vi "green_speedgate.vi"(4 "sat":cluster{"Lower value":i32, "Upper value":i32}={"Lower value"=30, "Upper value"=138}, 5 "luma":cluster{"Lower value":i32, "Upper value":i32}={"Lower value"=37, "Upper value"=106}, 6 "hue":cluster{"Lower value":i32, "Upper value":i32}={"Lower value"=80, "Upper value"=131}, 8 "error in (no error)":errorcluster, 11 "Image Src":T1) -> (0 "error out":errorcluster, 1 "max":dbl[](array[numeric]), 2 "green particles":dbl[][](array[numeric]), 3 "Image Out":T1(plugin-control))   [LabVIEW 2009]
uses:
  <vilib>/vision/Image Controls.llb/IMAQ Image.ctl
  <vilib>/vision/NI_Vision_Development_Module.lvlib
panel:
  out "Array":dbl[](array[numeric])
  out "Particle Measurements (Pixels)":dbl[][](array[numeric]) format="%.2f"
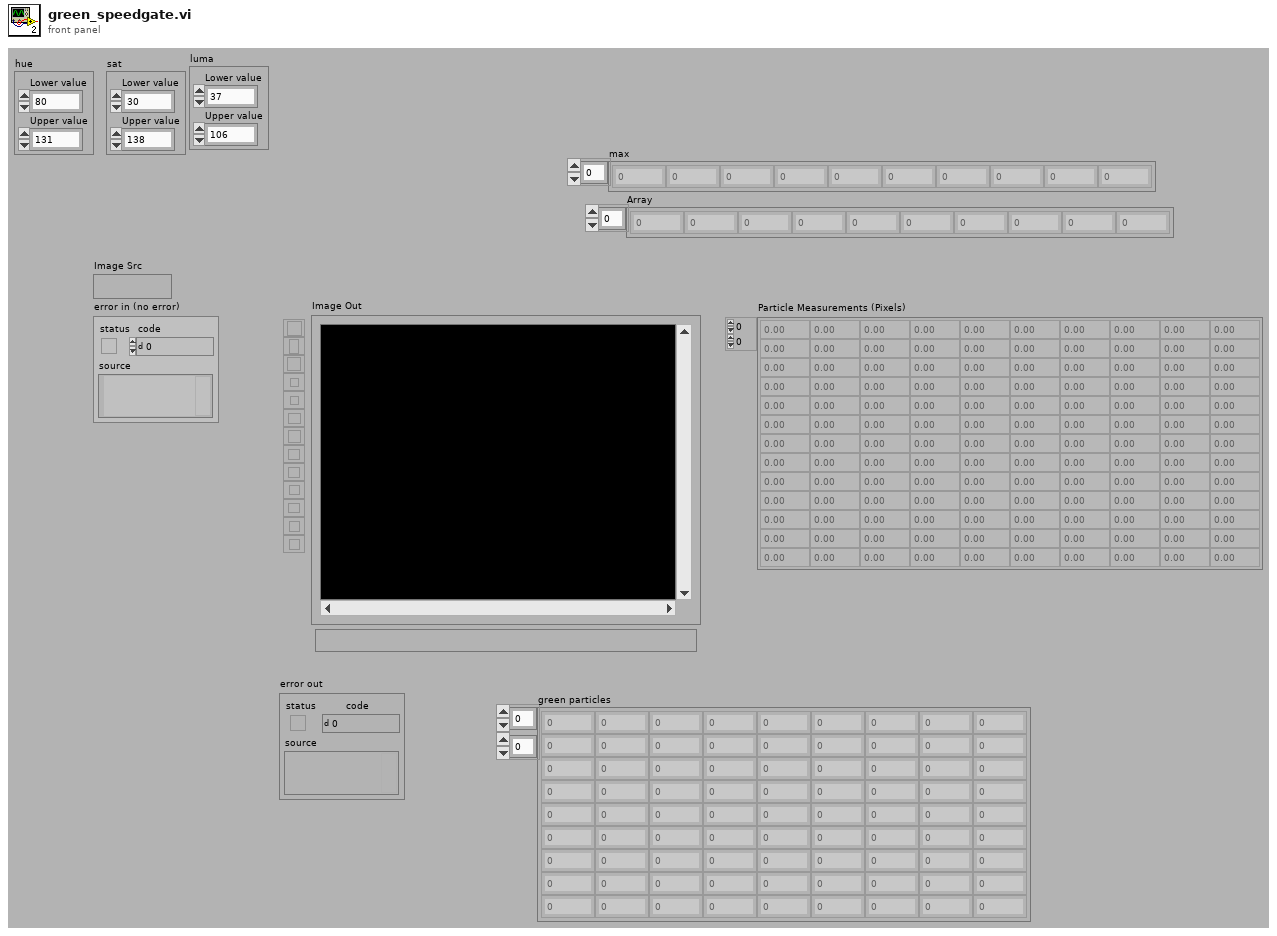
[diagram p1: front panel]
types:
  T1 = typedef "IMAQ Image.ctl" = refnum<image>
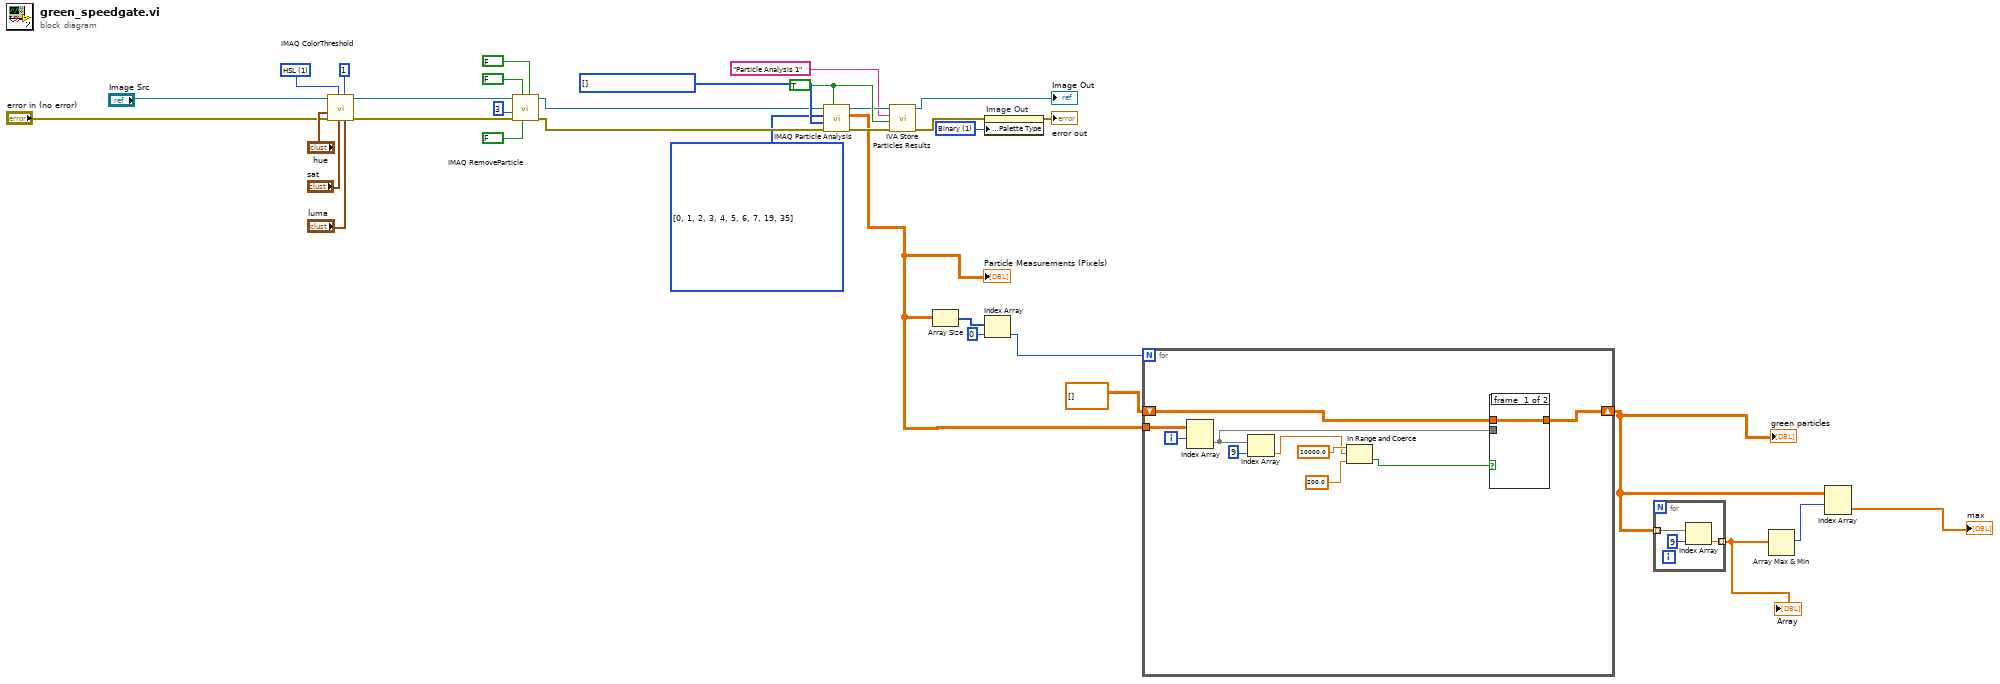
[diagram p0: block diagram]
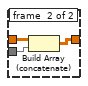
[diagram p2: hidden frame]
diagram:
  w19 = i32[] [] items=["Center of Mass X", "Center of Mass Y", "First Pixel X", "First Pixel Y", "Bounding Rect Left", "Bounding Rect Top", "Bounding Rect Right", "Bounding Rect Bottom", "Max Feret Diameter Start X", "Max Feret Diameter Start Y", "Max Feret Diameter End X", "Max Feret Diameter End Y", "Max Horiz. Segment Length Left", "Max Horiz. Segment Length Right", "Max Horiz. Segment Length Row", "-", "Bounding Rect Width", "Bounding Rect Height", "Bounding Rect Diagonal", "Perimeter", "Convex Hull Perimeter", "Holes' Perimeter", "Max Feret Diameter", "Equivalent Ellipse Major Axis", "Equivalent Ellipse Minor Axis", "Equivalent Ellipse Minor Axis (Feret)", "Equivalent Rect Long Side", "Equivalent Rect Short Side", "Equivalent Rect Diagonal", "Equivalent Rect Short Side (Feret)", "Average Horiz. Segment Length", "Average Vert. Segment Length", "Hydraulic Radius", "Waddel Disk Diameter", "-", "Area", "Holes' Area", "Particle & Holes' Area", "Convex Hull Area", "Image Area", "-", "Number of Holes", "Number of Horiz. Segments", "Number of Vert. Segments", "-", "Orientation", "Max Feret Diameter Orientation", "-", "% Area/Image Area", "% Area/(Particle & Holes' Area)", "Ratio of Equivalent Ellipse Axes", "Ratio of Equivalent Rect Sides", "-", "Elongation Factor", "Compactness Factor", "Heywood Circularity Factor", "Type Factor", "-", "Sum X", "Sum Y", "Sum XX", "Sum XY", "Sum YY", "Sum XXX", "Sum XXY", "Sum XYY", "Sum YYY", "-", "Moment of Inertia XX", "Moment of Inertia XY", "Moment of Inertia YY", "Moment of Inertia XXX", "Moment of Inertia XXY", "Moment of Inertia XYY", "Moment of Inertia YYY", "Norm. Moment of Inertia XX", "Norm. Moment of Inertia XY", "Norm. Moment of Inertia YY", "Norm. Moment of Inertia XXX", "Norm. Moment of Inertia XXY", "Norm. Moment of Inertia XYY", "Norm. Moment of Inertia YYY", "Hu Moment 1", "Hu Moment 2", "Hu Moment 3", "Hu Moment 4", "Hu Moment 5", "Hu Moment 6", "Hu Moment 7"] ("Real-World Measurements")
  w12 = i32[] [0, 1, 2, 3, 4, 5, 6, 7, 19, 35] items=["Center of Mass X", "Center of Mass Y", "First Pixel X", "First Pixel Y", "Bounding Rect Left", "Bounding Rect Top", "Bounding Rect Right", "Bounding Rect Bottom", "Max Feret Diameter Start X", "Max Feret Diameter Start Y", "Max Feret Diameter End X", "Max Feret Diameter End Y", "Max Horiz. Segment Length Left", "Max Horiz. Segment Length Right", "Max Horiz. Segment Length Row", "-", "Bounding Rect Width", "Bounding Rect Height", "Bounding Rect Diagonal", "Perimeter", "Convex Hull Perimeter", "Holes' Perimeter", "Max Feret Diameter", "Equivalent Ellipse Major Axis", "Equivalent Ellipse Minor Axis", "Equivalent Ellipse Minor Axis (Feret)", "Equivalent Rect Long Side", "Equivalent Rect Short Side", "Equivalent Rect Diagonal", "Equivalent Rect Short Side (Feret)", "Average Horiz. Segment Length", "Average Vert. Segment Length", "Hydraulic Radius", "Waddel Disk Diameter", "-", "Area", "Holes' Area", "Particle & Holes' Area", "Convex Hull Area", "Image Area", "-", "Number of Holes", "Number of Horiz. Segments", "Number of Vert. Segments", "-", "Orientation", "Max Feret Diameter Orientation", "-", "% Area/Image Area", "% Area/(Particle & Holes' Area)", "Ratio of Equivalent Ellipse Axes", "Ratio of Equivalent Rect Sides", "-", "Elongation Factor", "Compactness Factor", "Heywood Circularity Factor", "Type Factor", "-", "Sum X", "Sum Y", "Sum XX", "Sum XY", "Sum YY", "Sum XXX", "Sum XXY", "Sum XYY", "Sum YYY", "-", "Moment of Inertia XX", "Moment of Inertia XY", "Moment of Inertia YY", "Moment of Inertia XXX", "Moment of Inertia XXY", "Moment of Inertia XYY", "Moment of Inertia YYY", "Norm. Moment of Inertia XX", "Norm. Moment of Inertia XY", "Norm. Moment of Inertia YY", "Norm. Moment of Inertia XXX", "Norm. Moment of Inertia XXY", "Norm. Moment of Inertia XYY", "Norm. Moment of Inertia YYY", "Hu Moment 1", "Hu Moment 2", "Hu Moment 3", "Hu Moment 4", "Hu Moment 5", "Hu Moment 6", "Hu Moment 7"] ("Pixel Measurements")
  w18 = TRUE ("Connectivity 4/8 (8)")
  w23 = u32 1 items=["Grayscale", "Binary", "Gradient", "Rainbow", "Temperature", "User Defined"] ("Palette")
  w33 = u16 1 items=["RGB", "HSL", "HSV", "HSI"] ("Color Mode")
  n1 = call "IMAQ ColorThreshold"("Blue or Luma or Val or Inten Range"="luma", "Replace Value"=1, "Green or Sat Range"="sat", "Color Mode"=w33, "error in (no error)"="error in (no error)", "Red or Hue Range"="hue", "Image Src"="Image Src") -> ("error out"=w29:errorcluster, "Image Dst Out"=w24:T1)  [unwired: 1 in, 2 out]
  n2 = call "IMAQ RemoveParticle"("Connectivity 4/8 (8)"=FALSE, "Low Pass/High Pass (Low)"=FALSE, "Square/Hexa (Square)"=FALSE, "error in (no error)"=w29, "Number of Erosion"=3, "Image Src"=w24) -> ("error out"=w13:errorcluster, "Image Dst Out"=w14:T1)  [unwired: 1 in, 3 out]
  n3 = call "IMAQ Particle Analysis"("Connectivity 4/8 (8)"=w18, "error in (no error)"=w13, "Real-World Measurements"=w19, "Pixel Measurements"=w12, "Image"=w14) -> ("error out"=w15:errorcluster, "Particle Measurements (Pixels)"=w3:dbl[][], "Image Out (duplicate)"=w17:T1)  [unwired: 4 out]
  "Particle Measurements (Pixels)" <- w3
  n4 = call <vilib>:"IVA Store Particles Results.vi"("error in (no error)"=w15, "Connectivity 4/8 (8)"=w18, "Step Name"="Particle Analysis 1", "Image in"=w17) -> ("error out"=w1:errorcluster, "Image dup"=→"Image Out":T1)  [unwired: 6 out]
  n5 = Array Size(array=w3) -> (size(s)=w9:i32[])
  n6 = property on="Image Out" class="ImageControl"(error in=w1, "Palette:Palette Type"=w23) -> (error out=→"error out":errorcluster)  [unwired: 1 in, 1 out]
  n7 = Index Array(array=w9, index=0) -> (element=w11:i32)
  n8 = for {
    N: w11 -> [_]
    tunnel: w3 -> [w44]
    shift-right: [w39] -> w5
    shift-left: dbl[][] [] ("Particle Measurements (Pixels)") -> [w42]
    i -> [w43]
    n9 = Index Array(array=w44, index (row)=w43) -> (element=w40:dbl[])  [unwired: 1 in]
    n10 = Index Array(array=w40, index=9) -> (element=w36:dbl)
    n11 = In Range and Coerce(upper limit=10000.0, x=w36, lower limit=200.0) -> (In Range?=w35:bool)  [unwired: 1 out]
    n12 = case shown="True" w35 {
      tunnel: w42 -> [w45 w48]
      tunnel: w40 -> [_ w47]
      tunnel: [w45 w46] -> w39
      frame #0 {
      }
      frame #1 {
        n13 = Build Array (concatenate)(w48, w47) -> (w46:dbl[][])
      }
    }
  }
  "green particles" <- w5
  n14 = for {
    tunnel: [w50] -> w7 mode=indexing
    tunnel: w5 -> [w49] mode=indexing
    n15 = Index Array(array=w49, index=9) -> (element=w50:dbl)
  }
  "Array" <- w7
  n16 = Array Max & Min(array=w7) -> (max index (indices)=w6:i32)  [unwired: 3 out]
  n17 = Index Array(array=w5, index (row)=w6) -> (element=→"max":dbl[])  [unwired: 1 in]
